vi "read-write config ini path data.vi"(7 "Function":enum16{"Read", "Write"}(ring), 8 "error in (no error)":errorcluster, 10 "user data in":T1, 11 "file name":string) -> (0 "error out":errorcluster, 2 "user data out":T1)   [LabVIEW 2015]
doc: "This VI saves (Write) and retrieves (Read) data from a configuration .ini file, regardless of the number of sectors and the keys in each sector."
uses:
  <vilib>/Utility/config.llb/NI_LVConfig.lvlib
  <vilib>/Utility/config.llb/Read Key (String).vi
  <vilib>/Utility/config.llb/Write Key (String).vi
  controls/path data.ctl
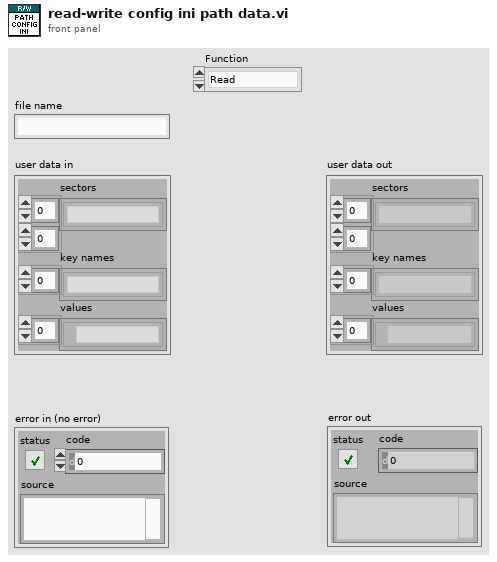
[diagram p1: front panel]
types:
  T1 = typedef "path data.ctl" = cluster{"sectors":string[][], "key names":string[], "values":path[]}
  T2 = typedef "NI_LVConfig.lvlib/Config Data RefNum.ctl" = refnum<k1>
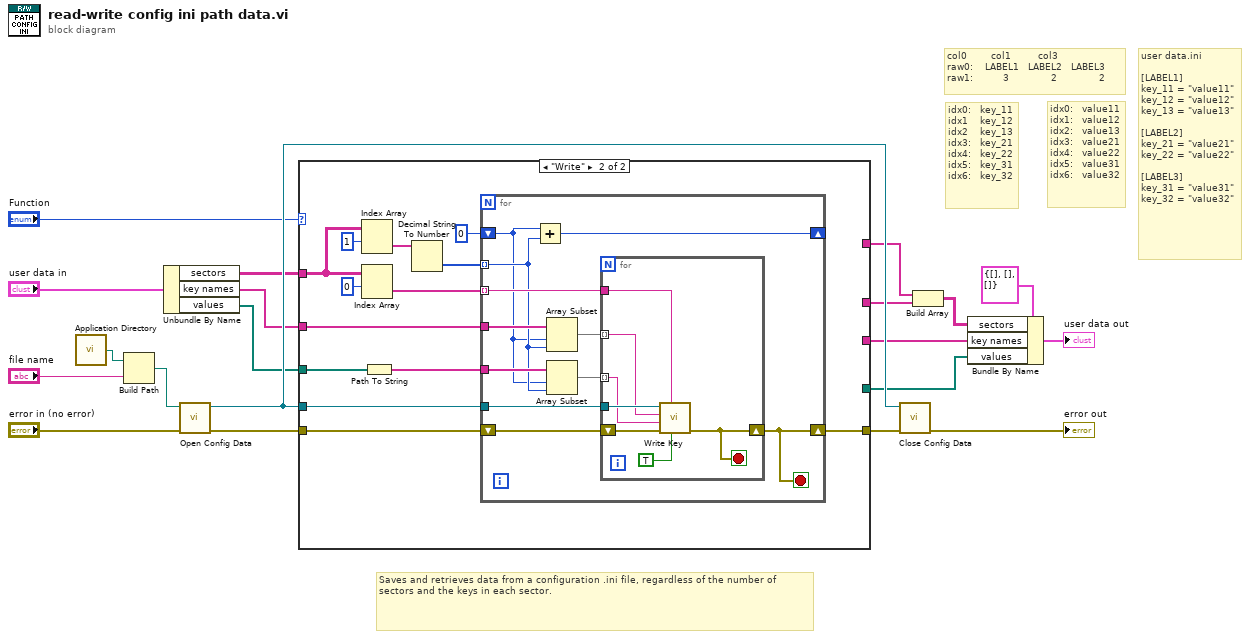
[diagram p0: block diagram]
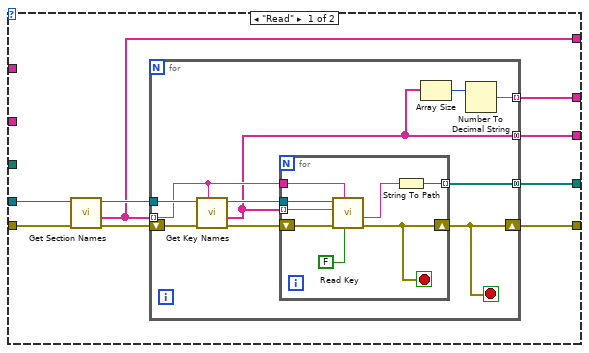
[diagram p2: hidden frame]
diagram:
  # "user data.ini\n\n[LABEL1]\nkey_11 = \"value11\"\nkey_12 = \"value12\"\nkey_13 = \"value13\"\n\n[LABEL2]\nkey_21 = \"value21\"\nkey_22 = \"value22\"\n\n[LABEL3]\nkey_31 = \"value31\"\nkey_32 = \"value32\""
  # "idx0:   value11\nidx1:   value12\nidx2:   value13\nidx3:   value21\nidx4:   value22\nidx5:   value31\nidx6:   value32"
  # "idx0:   key_11\nidx1    key_12\nidx2    key_13\nidx3:   key_21\nidx4:   key_22\nidx5:   key_31\nidx6:   key_32"
  # "col0        col1         col3   \nraw0:    LABEL1   LABEL2   LABEL3\nraw1:          3              2              2"
  # "Saves and retrieves data from a configuration .ini file, regardless of the number of sectors and the keys in each sector."
  n1 = call <vilib>:"Application Directory.vi"() -> ("Application Directory"=w16:path)
  n2 = Build Path(base path=w16, name or relative path="file name") -> (appended path=w18:path)
  n3 = Unbundle By Name("user data in") -> ("sectors"=w3:string[][], "key names"=w5:string[], "values"=w4:path[])
  n4 = call <vilib>:"Open Config Data.vi"("error in (no error)"="error in (no error)", "configuration file path"=w18) -> ("error out"=w20:errorcluster, "refnum"=w13:T2)  [unwired: 7 in, 1 out]
  n5 = case shown="\"Write\"" "Function" {
    tunnel: w20 -> [w27 w60]
    tunnel: [w26 w59] -> w15
    tunnel: w13 -> [w25 w57]
    tunnel: [w22 _] -> w9
    tunnel: [w24 _] -> w11
    tunnel: [w23 _] -> w10
    tunnel: w3 -> [_ w53]
    tunnel: w4 -> [_ w58]
    tunnel: w5 -> [_ w49]
    tunnel: [w21 _] -> w8
    frame "Read" {
      n6 = call <vilib>:"Get Section Names.vi"("error in (no error)"=w27, "refnum"=w25) -> ("error out"=w28:errorcluster, "section names"=w22:string[], "refnum out"=w29:T2)  [unwired: 7 in]
      n7 = for {
        tunnel: w29 -> [w39]
        tunnel: w22 -> [w33] mode=indexing
        shift-right: [w35] -> w26
        shift-left: w28 -> [w38]
        tunnel: [w32] -> w24 mode=concatenating
        tunnel: [w34] -> w23 mode=concatenating
        tunnel: [w30] -> w21 mode=indexing
        stop <- w35 stop-if-true
        n8 = call <vilib>:"Get Key Names.vi"("section"=w33, "error in (no error)"=w38, "refnum"=w39) -> ("error out"=w37:errorcluster, "key names"=w32:string[], "refnum out"=w36:T2)  [unwired: 5 in, 1 out]
        n9 = for {
          shift-right: [w42] -> w35
          shift-left: w37 -> [w47]
          tunnel: w32 -> [w43] mode=indexing
          tunnel: w36 -> [w46]
          tunnel: w33 -> [w45]
          tunnel: [w40] -> w34 mode=indexing
          stop <- w42 stop-if-true
          n10 = call-poly <vilib>:"Read Key.vi"("read raw string? (F)"=FALSE, "section"=w45, "error in (no error)"=w47, "key"=w43, "refnum"=w46) -> ("error out"=w42:errorcluster, "value"=w44:string)  [unwired: 3 in, 2 out]
          n11 = String To Path(string=w44) -> (path=w40:path)
        }
        n12 = Array Size(array=w32) -> (size(s)=w31:i32)
        n13 = Number To Decimal String(number=w31) -> (decimal integer string=w30:string)  [unwired: 1 in]
      }
    }
    frame "Write" {
      n14 = Index Array(array=w53, index (row)=1) -> (element=w52:string[])  [unwired: 1 in]
      n15 = Index Array(array=w53, index (row)=0) -> (element=w55:string[])  [unwired: 1 in]
      n16 = Path To String(path=w58) -> (string=w48:string[])
      n17 = Decimal String To Number(string=w52) -> (number=w51:i32[])  [unwired: 2 in, 1 out]
      n18 = for {
        tunnel: w48 -> [w64]
        tunnel: w49 -> [w67]
        tunnel: w57 -> [w70]
        tunnel: w55 -> [w69] mode=indexing
        shift-right: [w68] -> w59
        shift-left: w60 -> [w71]
        tunnel: w51 -> [w62] mode=indexing
        shift-right: [w65] -> _
        shift-left: 0 ("sector") -> [w61]
        stop <- w68 stop-if-true
        n19 = Add(x=w61, y=w62) -> (x+y=w65:i32)
        n20 = Array Subset(array=w67, index=w61, length=w62) -> (w66:string[])
        n21 = Array Subset(array=w64, index=w61, length=w62) -> (w63:string[])
        n22 = for {
          tunnel: w70 -> [w78]
          shift-right: [w73] -> w68
          shift-left: w71 -> [w77]
          tunnel: w69 -> [w76]
          tunnel: w66 -> [w75] mode=indexing
          tunnel: w63 -> [w74] mode=indexing
          stop <- w73 stop-if-true
          n23 = call-poly <vilib>:"Write Key.vi"("write raw string? (F)"=TRUE, "section"=w76, "error in (no error)"=w77, "value"=w74, "key"=w75, "refnum"=w78) -> ("error out"=w73:errorcluster)  [unwired: 3 in, 2 out]
        }
      }
    }
  }
  n24 = call <vilib>:"Close Config Data.vi"("error in (no error)"=w15, "refnum"=w13) -> ("error out"=→"error out":errorcluster)  [unwired: 8 in, 1 out]
  n25 = Build Array(w9, w8) -> (w7:string[][])
  n26 = Bundle By Name(cluster=T1 {"sectors"=[], "key names"=[], "values"=[]} ("user data out"), "sectors"=w7, "key names"=w11, "values"=w10) -> (→"user data out":T1)
